vi "Advantech Setup Channels.vi"(8 "error in (no error)":errorcluster) -> (0 "error out":errorcluster, 3 "task out":i32)   [LabVIEW 2018]
uses:
  <userlib>/DAQNavi Polymorphic VI/configure/DAQNavi Get Property/Device/DAQNaviGet_Device_SupportedDevices.vi
  <userlib>/DAQNavi Polymorphic VI/create/DAQNavi Create Channel(AI-Current).vi
  <userlib>/DAQNavi Polymorphic VI/create/DAQNavi Create Channel(AI-Temperature).vi
  <userlib>/DAQNavi Polymorphic VI/create/DAQNavi Create Channel(AI-Voltage).vi
panel:
  out "supported devices":string[](array[string])
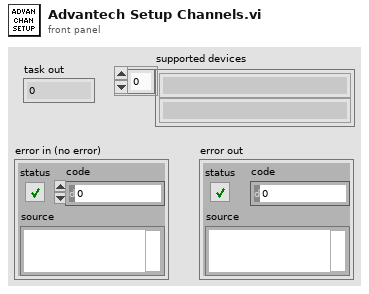
[diagram p1: front panel]
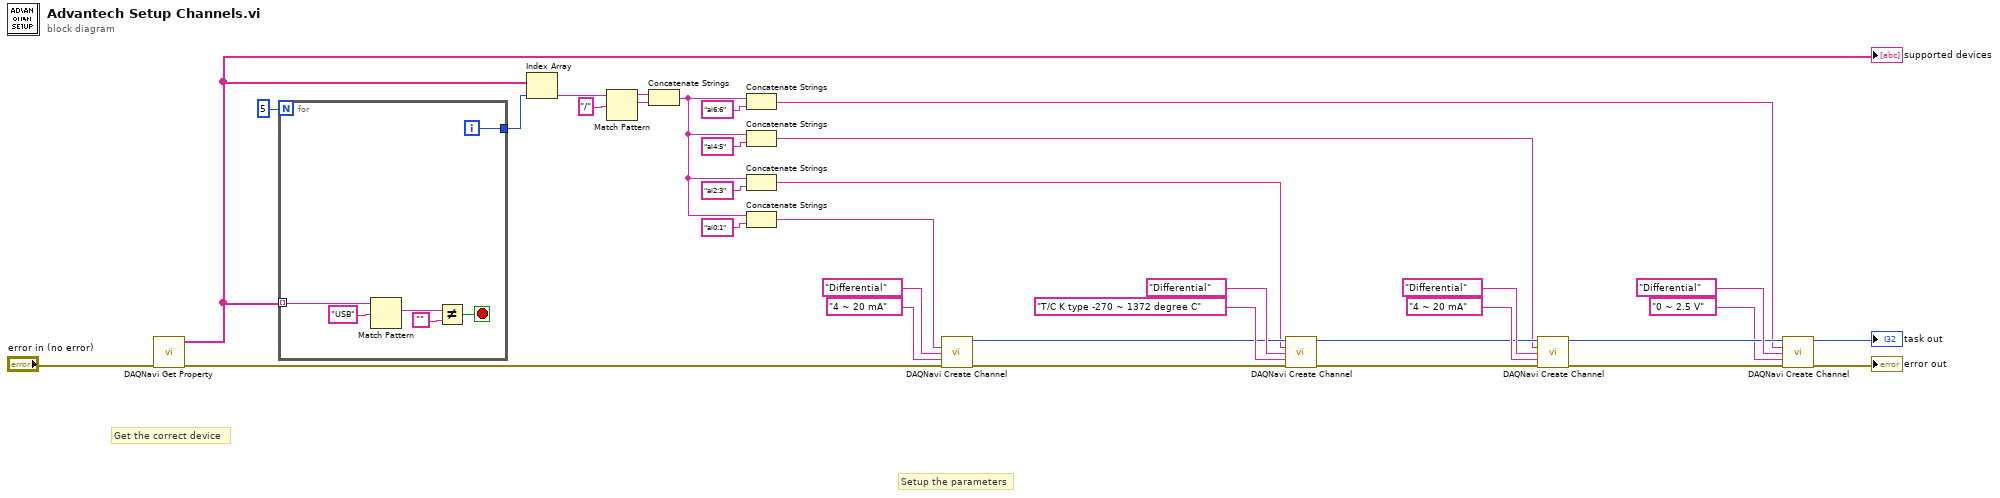
[diagram p0: block diagram]
diagram:
  # "Setup the parameters"
  # "Get the correct device"
  n1 = call-poly <userlib>:"DAQNavi Get Property.vi"("error in (no error)"="error in (no error)") -> ("error out"=w14:errorcluster, "supported devices"=w3:string[])  [unwired: 9 in]
  "supported devices" <- w3
  n2 = for {
    N: 5 -> [_]
    tunnel: w3 -> [w40] mode=indexing
    tunnel: [w38] -> w1
    i -> [w38]
    stop <- w36 stop-if-true
    n3 = Match Pattern(string=w40, regular expression="USB") -> (match substring=w35:string)  [unwired: 1 in, 3 out]
    n4 = Not Equal?(x=w35, y="") -> (x != y?=w36:bool)
  }
  n5 = Index Array(array=w3, index=w1) -> (element=w18:string)
  n6 = Match Pattern(string=w18, regular expression="/") -> (before substring=w16:string, match substring=w15:string)  [unwired: 1 in, 2 out]
  n7 = Concatenate Strings(w16, w15) -> (w7:string)
  n8 = Concatenate Strings(w7, "ai6:6") -> (w6:string)
  n9 = Concatenate Strings(w7, "ai4:5") -> (w5:string)
  n10 = Concatenate Strings(w7, "ai2:3") -> (w10:string)
  n11 = Concatenate Strings(w7, "ai0:1") -> (w12:string)
  n12 = call-poly <userlib>:"DAQNavi Create Channel.vi"("physical channels"=w12, "signal type"="Differential", "value range"="4 ~ 20 mA", "error in (no error)"=w14) -> ("task out"=w22:i32, "error out"=w32:errorcluster)  [unwired: 10 in]
  n13 = call-poly <userlib>:"DAQNavi Create Channel.vi"("task in"=w22, "physical channels"=w10, "signal type"="Differential", "value range"="T/C K type -270 ~ 1372 degree C", "error in (no error)"=w32) -> ("task out"=w25:i32, "error out"=w31:errorcluster)  [unwired: 9 in]
  n14 = call-poly <userlib>:"DAQNavi Create Channel.vi"("task in"=w25, "physical channels"=w5, "signal type"="Differential", "value range"="4 ~ 20 mA", "error in (no error)"=w31) -> ("task out"=w28:i32, "error out"=w30:errorcluster)  [unwired: 9 in]
  n15 = call-poly <userlib>:"DAQNavi Create Channel.vi"("task in"=w28, "physical channels"=w6, "signal type"="Differential", "value range"="0 ~ 2.5 V", "error in (no error)"=w30) -> ("task out"=→"task out":i32, "error out"=→"error out":errorcluster)  [unwired: 9 in]
